vi "MoveByTextInFileName.vi"() -> ()   [LabVIEW 2011]
uses:
  <vilib>/Utility/file.llb/Read From Spreadsheet File (string).vi
panel:
  in  "OK Button":bool
  out "Errors":errorcluster[](array[cluster])
  in  "target path (use dialog)":path
  in  "pattern":string
  in  "directory to find text":path
  in  "delimiter (\\t)":string="\t"
  in  "List of string values":path
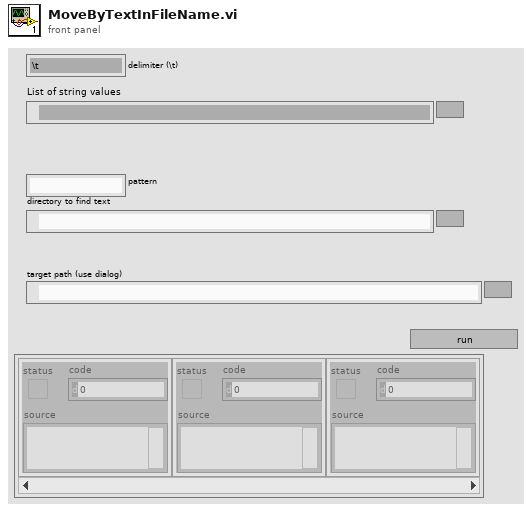
[diagram p1: front panel]
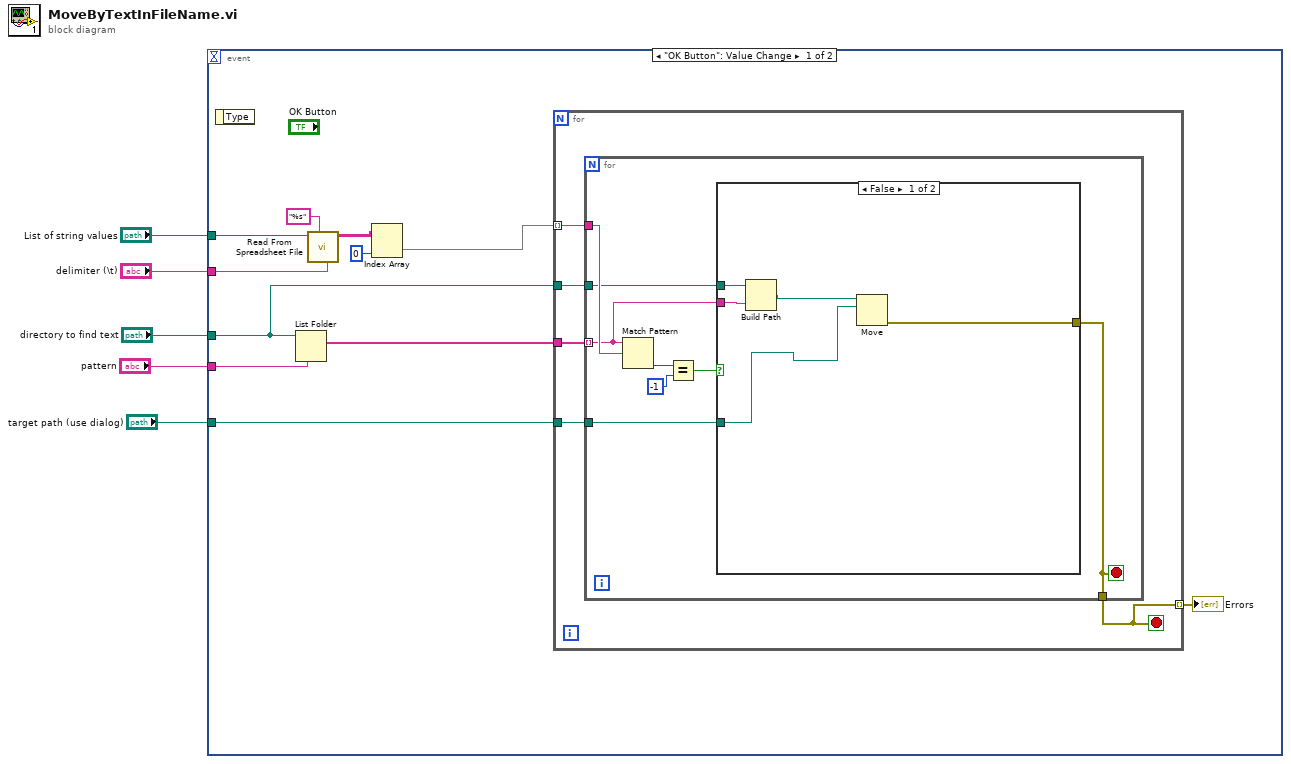
[diagram p0: block diagram]
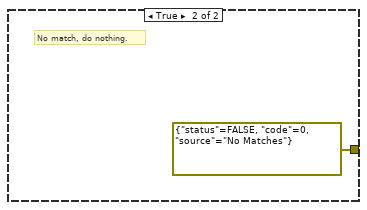
[diagram p2: hidden frame]
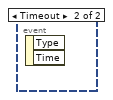
[diagram p3: hidden frame]
diagram:
  n1 = event shown="[0] \"OK Button\": Value Change" {
    selector: _ -> [_ _]
    dyn-events: _ -> [_ _]
    timeout: _ -> [_ _]
    tunnel: "List of string values" -> [w16 _]
    tunnel: "delimiter (\\t)" -> [w7 _]
    tunnel: "pattern" -> [w12 _]
    tunnel: "directory to find text" -> [w10 _]
    tunnel: "target path (use dialog)" -> [w9 _]
    event "OK Button": Value Change {
      n2 = event-data() -> ()  [unwired: 1 in, 1 out]
      n3 = List Folder(path=w10, pattern=w12) -> (filenames=w11:string[])  [unwired: 2 in, 3 out]
      n4 = call-poly <vilib>:"Read From Spreadsheet File.vi"("delimiter (\\t)"=w7, "format (%s)"="%s" ("format (%.3f)"), "file path (dialog if empty)"=w16) -> ("all rows"=w14:string[][])  [unwired: 4 in, 4 out]
      n5 = Index Array(array=w14, index (col)=0 ("disabled index (col)")) -> (element=w6:string[])  [unwired: 1 in]
      n6 = for {
        tunnel: w6 -> [w20] mode=indexing
        tunnel: w11 -> [w21]
        tunnel: w10 -> [w19]
        tunnel: w9 -> [w18]
        tunnel: [w17] -> w8 mode=indexing
        stop <- w17 stop-if-true
        n7 = for {
          tunnel: w21 -> [w24] mode=indexing
          tunnel: w20 -> [w29]
          tunnel: w19 -> [w25]
          tunnel: w18 -> [w23]
          tunnel: [w22] -> w17
          stop <- w22 stop-if-true
          n8 = Match Pattern(string=w24, regular expression=w29) -> (offset past match=w28:i32)  [unwired: 1 in, 3 out]
          n9 = Equal?(x=w28, y=-1) -> (x = y?=w26:bool)
          n10 = case shown="False" w26 {
            tunnel: w25 -> [w34 _]
            tunnel: w24 -> [w31 _]
            tunnel: w23 -> [w30 _]
            tunnel: [w32 errorcluster {"status"=FALSE, "code"=0, "source"="No Matches"} ("error out")] -> w22
            frame False {
              n11 = Build Path(base path=w34, name or relative path=w31) -> (appended path=w33:path)
              n12 = Move(source path=w33, 10:w30) -> (error out=w32:errorcluster)  [unwired: 3 in, 2 out]
            }
            frame True {
              # "No match, do nothing."
            }
          }
        }
      }
      "Errors" <- w8
    }
    event Timeout {
      n13 = event-data() -> ()  [unwired: 1 in, 2 out]
    }
  }
